vi "RPM to Radians per Second.vi"   [LabVIEW 2017, in "NI_Robotics Utilities.lvlib"]
doc: "Converts an angular velocity from rpm to radians per second."
uses:
  <vilib>/robotics/Utilities/NI_Robotics Utilities.lvlib
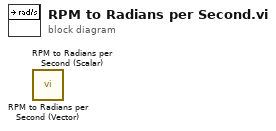
[diagram p0: block diagram]
diagram:
  n1 = call <vilib>:"RPM to Radians per Second (Vector).vi"() -> ()  [unwired: 3 in, 1 out]
  n2 = call <vilib>:"RPM to Radians per Second (Scalar).vi"() -> ()  [unwired: 3 in, 1 out]
